vi "niRFUtil MT UTIL IQ Impairments DC Offset.vi"(0 "Waveform In":T1={"x0"=0.0, "dx"=1.0, "y"=[]} caption="input complex waveform" {"y" format="%.2f"; "dx" format="%^.2e"; "x0" format="%^.2e"}, 1 "I DC Offset, %":dbl format="%.2f", 2 "Q DC Offset, %":dbl format="%.2f", 5 "Gain Scaling factor":dbl, 11 "error in (no error)":errorcluster) -> (4 "Waveform Out":T1 caption="output complex waveform" {"y" format="%.2f"; "dx" format="%^.2e"; "x0" format="%^.2e"}, 15 "error out":errorcluster)   [LabVIEW 2015, in "niRFUtil.lvlib"]
doc: "Performs the DC Offset operation for IQ Impairment of an Input Data Waveform."
uses:
  niRFUtil.lvlib
  Includes/niRFUtil INC Complex Waveform.ctl
  Includes/niRFUtil INC Complex Array.ctl
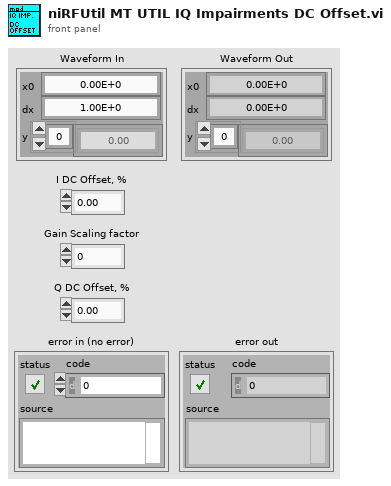
[diagram p1: front panel]
types:
  T1 = typedef "niRFUtil.lvlib/niRFUtil INC Complex Waveform.ctl" = cluster{"x0":dbl, "dx":dbl, "y":T2}
  T2 = typedef "niRFUtil.lvlib/niRFUtil INC Complex Array.ctl" = csg[]
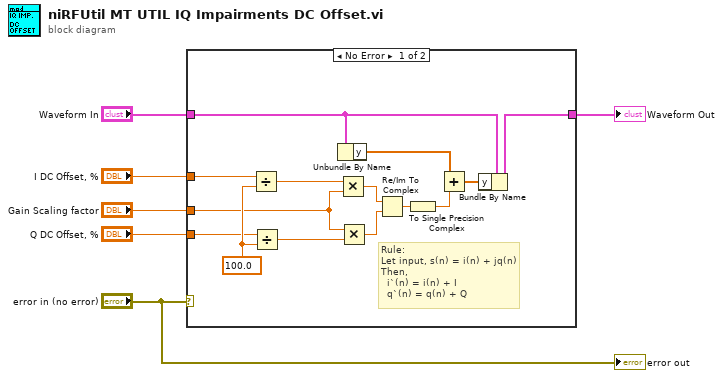
[diagram p0: block diagram]
diagram:
  n1 = case shown="No Error" "error in (no error)" {
    tunnel: "I DC Offset, %" -> [w10 _]
    tunnel: "Q DC Offset, %" -> [w9 _]
    tunnel: "Waveform In" -> [w12 w21]
    tunnel: [w11 w21] -> w3
    tunnel: "Gain Scaling factor" -> [w8 _]
    frame No Error {
      w20 = 100.0 ("y")
      # "Rule:\nLet input, s(n) = i(n) + jq(n)\nThen,\n  i`(n) = i(n) + I\n  q`(n) = q(n) + Q"
      n2 = Divide(x=w10, y=w20) -> (x/y=w18:dbl)
      n3 = Divide(x=w9, y=w20) -> (x/y=w19:dbl)
      n4 = Unbundle By Name(w12) -> ("y"=w13:T2)
      n5 = Multiply(x=w18, y=w8) -> (x*y=w16:dbl)
      n6 = Multiply(x=w8, y=w19) -> (x*y=w15:dbl)
      n7 = Re/Im To Complex(1:w15, 2:w16) -> (0:w17:cdb)
      n8 = To Single Precision Complex(1:w17) -> (0:w7:csg)
      n9 = Add(x=w13, y=w7) -> (x+y=w14:T2)
      n10 = Bundle By Name(cluster=w12, "y"=w14) -> (w11:T1)
    }
    frame Error {
    }
  }
  "Waveform Out" <- w3
  "error out" <- "error in (no error)"
